vi "Test.vi"() -> ()   [LabVIEW 2019]
uses:
  VoiceCommandState.ctl
  <vilib>/myRIO/Instrument Drivers/Onboard IO/DIO/typedefs/DIO Reference.ctl
  <vilib>/myRIO/Common/Instrument Driver Framework/Utilities/typedefs/myRIO Generic Hardware Reference.ctl
  <vilib>/myRIO/Common/Instrument Driver Framework/Utilities/typedefs/Hardware Version Enum.ctl
  <vilib>/myRIO/Common/Instrument Driver Framework/Utilities/typedefs/myRIO v1.0 Reference.ctl
  <vilib>/myRIO/Common/Instrument Driver Framework/Utilities/typedefs/Generic FPGA Reference.ctl
  <vilib>/myRIO/Common/Instrument Driver Framework/myRIO v1.0/DIO/typedefs/DIO Channels List.ctl
  <vilib>/myRIO/Common/Instrument Driver Framework/myRIO v1.0/DIO/typedefs/DIO Channels Enum.ctl
  <vilib>/userDefined/High Color/nirio_resource_hc.ctl
  <vilib>/myRIO/Common/Instrument Driver Framework/Utilities/vis/Is FPGA Ref Available.vi
  <vilib>/myRIO/Common/Instrument Driver Framework/myRIO v1.0/DIO/vis/myRIO v1.1 Open DIO.vi
  <vilib>/myRIO/Common/Instrument Driver Framework/Utilities/vis/Validate Channels.vi
  <vilib>/myRIO/Common/Instrument Driver Framework/myRIO v1.0/DIO/vis/myRIO v1.0 Reserve DIO.vi
  <vilib>/myRIO/Common/Instrument Driver Framework/myRIO v1.0/UART/vis/myRIO v1.0 Close UART.vi
  <vilib>/myRIO/Common/Instrument Driver Framework/myRIO v1.0/Resource Manager/vis/myRIO v1.0 Reserve Channel List.vi
  <vilib>/myRIO/Common/Instrument Driver Framework/myRIO v1.0/DIO/vis/myRIO v1.0 Build MUX Configuration DIO.vi
  <vilib>/myRIO/Common/Instrument Driver Framework/myRIO v1.0/Resource Manager/vis/myRIO v1.0 Reserve Channel.vi
  <vilib>/myRIO/Common/Instrument Driver Framework/myRIO v1.0/Resource Manager/vis/myRIO v1.0 Unreserve Channel.vi
  <vilib>/myRIO/Common/Instrument Driver Framework/myRIO v1.0/Resource Manager/vis/myRIO v1.0 Create Configuration List.vi
  <vilib>/myRIO/Common/Instrument Driver Framework/myRIO v1.0/Resource Manager/vis/myRIO v1.0 Build Mutex Name.vi
  <vilib>/Utility/VariantDataType/GetNumericInfo.vi
  <vilib>/Utility/error.llb/Error Cluster From Error Code.vi
  <vilib>/myRIO/Common/Instrument Driver Framework/myRIO v1.0/myRIO v1.1 Open.vi
  <vilib>/myRIO/Common/Instrument Driver Framework/Utilities/vis/IO Manager.vi
  <vilib>/myRIO/Common/Instrument Driver Framework/Utilities/vis/Configuration Manager.vi
  <vilib>/myRIO/Common/Instrument Driver Framework/myRIO v1.0/Resource Manager/vis/myRIO v1.0 Configure IO.vi
  <vilib>/myRIO/Common/Instrument Driver Framework/myRIO v1.0/myRIO v1.0 Close.vi
  <vilib>/myRIO/Common/Instrument Driver Framework/myRIO v1.0/DIO/vis/myRIO v1.0 Write DIO.vi
  <vilib>/myRIO/Common/Instrument Driver Framework/Utilities/vis/FPGA Ref Manager.vi
  <vilib>/myRIO/Common/Instrument Driver Framework/myRIO v1.0/myRIO v1.0 Reset FPGA.vi
  <vilib>/myRIO/Common/Instrument Driver Framework/myRIO v1.0/IRQ/vis/myRIO v1.0 IRQ Info FGV.vi
  <vilib>/myRIO/Common/Instrument Driver Framework/myRIO v1.0/IRQ/vis/myRIO v1.0 Timer IRQ Info FGV.vi
  <vilib>/myRIO/Common/Instrument Driver Framework/myRIO v1.0/IRQ/vis/myRIO v1.0 ISR Agent.vi
  <vilib>/myRIO/Instrument Drivers/Utilities/vis/Reset Index.vi
  <vilib>/myRIO/Common/Instrument Driver Framework/myRIO v1.0/Resource Manager/vis/myRIO v1.0 Block Write Resource Manager.vi
  <vilib>/myRIO/Express VI/Onboard IO/DO/DO Express VI.xnode
  <vilib>/myRIO/Instrument Drivers/Onboard IO/DIO/vis/myRIO DIO Open.xnode
  Downloads/builds/DFRobot_ASR_myRIO_Lib/myRIO-1900/DFR_ISRM_myRIO/home/lvuser/natinst/bin/DFR_ISRM_myRIO.lvlibp
  Simple Queue Message/Simple Queue Message.lvlib
  <vilib>/myRIO/Instrument Drivers/Onboard IO/DIO/DIO.lvlib
  <vilib>/myRIO/Instrument Drivers/Utilities/Utilities.lvlib
panel:
  out "appended array 2":T1[](array[typedef])
  out "concatenated string":string
  out "String":string
  out "State":T1
  out "appended array":i32[](array[numeric])
  out "Result History":i32[](array[numeric])
  in  "Stop Button":bool
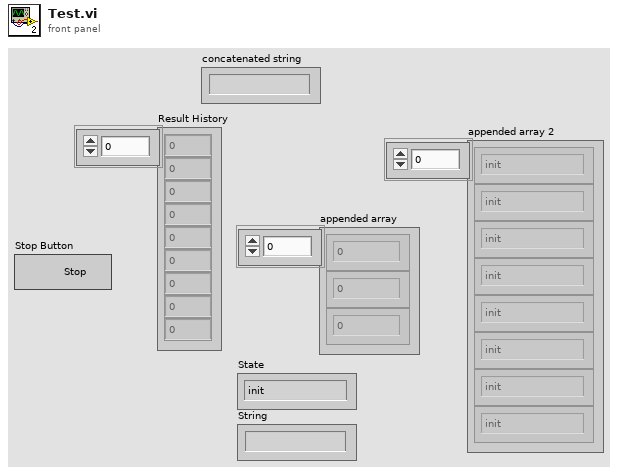
[diagram p1: front panel]
types:
  T1 = typedef "VoiceCommandState.ctl" = enum16{"init", "command", "quantity", "finish", "err"}
  T2 = typedef "DIO.lvlib/DIO Reference.ctl" = cluster{"myRIO Reference":T3, "DIO Channels List":T7}
  T3 = typedef "myRIO Generic Hardware Reference.ctl" = cluster{"myRIO Model":T4, "myRIO Hardware Reference":T5}
  T4 = typedef "Hardware Version Enum.ctl" = enum16{"Unknown", "myRIO-1900", "myRIO-1950", "roboRIO", "NI ELVIS RIO CM", "ELVIS III"}
  T5 = typedef "myRIO v1.0 Reference.ctl" = cluster{"Generic FPGA Reference":T6, "Allow multiple opens":bool}
  T6 = typedef "Generic FPGA Reference.ctl" = refnum<k20>
  T7 = typedef "DIO Channels List.ctl" = T8[]
  T8 = typedef "DIO Channels Enum.ctl" = enum16{"Not Connected", "C/DIO0", "C/DIO1", "C/DIO2", "C/DIO3", "C/DIO4", "C/DIO5", "C/DIO6", "C/DIO7", "A/DIO0", "A/DIO1", "A/DIO2", "A/DIO3", "A/DIO4", "A/DIO5", "A/DIO6", "A/DIO7", "A/DIO8", "A/DIO9", "A/DIO10", "A/DIO11", "A/DIO12", "A/DIO13", "A/DIO14", "A/DIO15", "A/DIO16", "A/DIO17", "A/DIO18", "A/DIO19", "B/DIO0", "B/DIO1", "B/DIO2", "B/DIO3", "B/DIO4", "B/DIO5", "B/DIO6", "B/DIO7", "B/DIO8", "B/DIO9", "B/DIO10", "B/DIO11", "B/DIO12", "B/DIO13", "B/DIO14", "B/DIO15", "B/DIO16", "B/DIO17", "B/DIO18", "B/DIO19", "LED0", "LED1", "LED2", "LED3", "Button0", "DIO/DIO0", "DIO/DIO1", "DIO/DIO2", "DIO/DIO3", "DIO/DIO4", "DIO/DIO5", "DIO/DIO6", "DIO/DIO7", "DIO/DIO8", "DIO/DIO9", "SPI/CS0", "SPI/CS1", "SPI/CS2", "SPI/CS3", "LED RADIO (Green)", "LED RADIO (Red)", "LED COMM (Green)", "LED COMM (Red)", "LED MODE (Green)", "LED MODE (Red)"}
  T9 = typedef "nirio_resource_hc.ctl" = tag
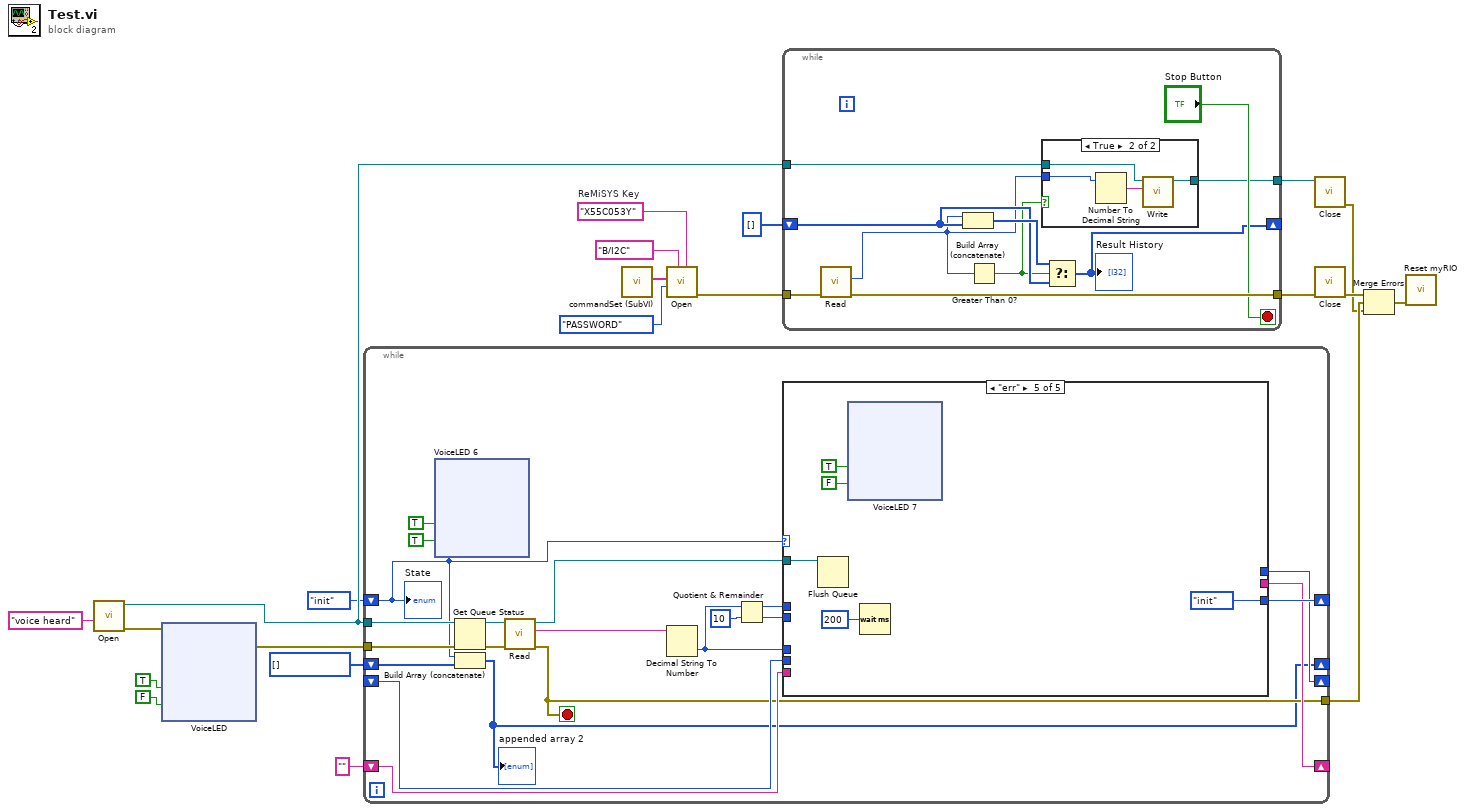
[diagram p0: block diagram]
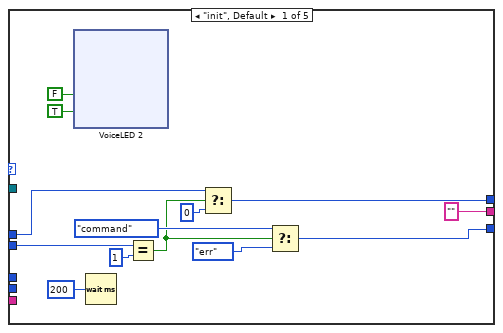
[diagram p2: hidden frame]
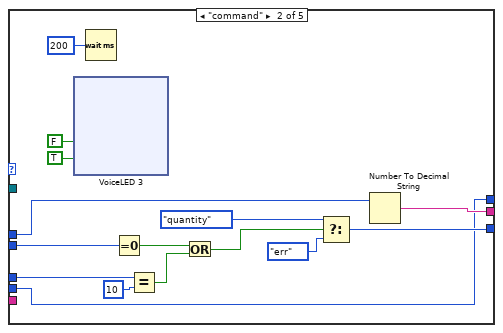
[diagram p3: hidden frame]
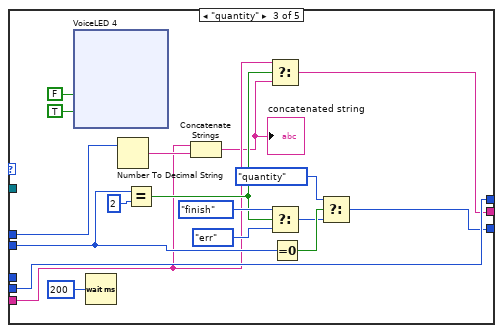
[diagram p4: hidden frame]
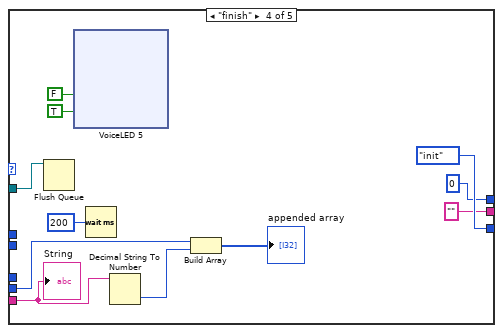
[diagram p5: hidden frame]
diagram:
  w2 = T1[] [] items=["init", "command", "quantity", "finish", "err"]
  w21 = "X55C053Y"  # ReMiSYS Key
  n1 = call "Open.vi"("name (unnamed)"="voice heard") -> ("error out"=w8:errorcluster, "queue out"=w13:refnum<queue>)  [unwired: 9 in]
  n2 = xnode "VoiceLED"("Green (C/DIO6 (DIO6))"=TRUE, "Red (C/DIO7 (DIO7))"=FALSE, "error in (no error)"=w8) -> ("error out"=w11:errorcluster)
  n3 = while {
    tunnel: w13 -> [w32]
    shift-right: [w41] -> _
    shift-left: VoiceCommandState."init" -> [w27]
    shift-right: [w38] -> _
    shift-left: "" -> [w37]
    tunnel: w11 -> [w30]
    shift-right: [w35] -> _
    shift-left: _ -> [w34]
    tunnel: [w28] -> w4
    shift-right: [w26] -> _
    shift-left: w2 -> [w25]
    stop <- w28 stop-if-true
    n4 = xnode "VoiceLED 6"("Green (C/DIO6 (DIO6))"=TRUE, "Red (C/DIO7 (DIO7))"=TRUE) -> ()  [unwired: 1 in, 1 out]
    n5 = Get Queue Status(queue=w32, error in (no error)=w30) -> (queue out=w31:refnum<queue>, error out=w29:errorcluster)  [unwired: 1 in, 6 out]
    n6 = Build Array (concatenate)(w27, w25) -> (w26:T1[])
    "appended array 2" <- w26
    n7 = call "Read.vi"("error in (no error)"=w29, "queue"=w31) -> ("error out"=w28:errorcluster, "state"=w42:string, "queue out"=w33:refnum<queue>)  [unwired: 6 in, 1 out]
    n8 = Decimal String To Number(string=w42) -> (number=w24:i32)  [unwired: 2 in, 1 out]
    n9 = Quotient & Remainder(x=w24, y=10) -> (x-y*floor(x/y)=w36:i32, floor(x/y)=w39:i32)
    n10 = case shown="\"err\"" w27 {
      tunnel: [w88 w142 w185 VoiceCommandState."init" VoiceCommandState."init"] -> w41
      tunnel: w39 -> [w87 w135 w193 _ _]
      tunnel: ["" w139 w181 "" _] -> w38
      tunnel: w37 -> [_ _ w183 w242 _]
      tunnel: [w82 w136 w186 0 ("f") _] -> w35
      tunnel: w36 -> [w83 w134 w180 _ _]
      tunnel: w34 -> [_ w136 w186 w243 _]
      tunnel: w33 -> [_ _ _ w234 w284]
      tunnel: w24 -> [_ w132 _ _ _]
      frame "init", Default {
        n11 = xnode "VoiceLED 2"("Green (C/DIO6 (DIO6))"=FALSE, "Red (C/DIO7 (DIO7))"=TRUE) -> ()  [unwired: 1 in, 1 out]
        n12 = Wait (ms)(milliseconds to wait=u32 200) -> ()  [unwired: 1 out]
        n13 = Equal?(x=w87, y=1) -> (x = y?=w84:bool)
        n14 = Select(t=w83, s=w84, f=0) -> (s? t:f=w82:i32)
        n15 = Select(t=VoiceCommandState."command", s=w84, f=VoiceCommandState."err") -> (s? t:f=w88:T1)
      }
      frame "command" {
        n16 = xnode "VoiceLED 3"("Green (C/DIO6 (DIO6))"=FALSE, "Red (C/DIO7 (DIO7))"=TRUE) -> ()  [unwired: 1 in, 1 out]
        n17 = Wait (ms)(milliseconds to wait=u32 200) -> ()  [unwired: 1 out]
        n18 = Equal To 0?(x=w135) -> (x = 0?=w133:bool)
        n19 = Equal?(x=w132, y=10) -> (x = y?=w130:bool)
        n20 = Or(x=w133, y=w130) -> (x .or. y?=w129:bool)
        n21 = Select(t=VoiceCommandState."quantity", s=w129, f=VoiceCommandState."err") -> (s? t:f=w142:T1)
        n22 = Number To Decimal String(number=w134) -> (decimal integer string=w139:string)  [unwired: 1 in]
      }
      frame "quantity" {
        n23 = xnode "VoiceLED 4"("Green (C/DIO6 (DIO6))"=FALSE, "Red (C/DIO7 (DIO7))"=TRUE) -> ()  [unwired: 1 in, 1 out]
        n24 = Wait (ms)(milliseconds to wait=u32 200) -> ()  [unwired: 1 out]
        n25 = Number To Decimal String(number=w180) -> (decimal integer string=w196:string)  [unwired: 1 in]
        n26 = Equal?(x=w193, y=2) -> (x = y?=w184:bool)
        n27 = Concatenate Strings(w183, w196) -> (w182:string)
        "concatenated string" <- w182
        n28 = Select(t=w183, s=w184, f=w182) -> (s? t:f=w181:string)
        n29 = Select(t=VoiceCommandState."finish", s=w184, f=VoiceCommandState."err") -> (s? t:f=w188:T1)
        n30 = Equal To 0?(x=w193) -> (x = 0?=w195:bool)
        n31 = Select(t=VoiceCommandState."quantity", s=w195, f=w188) -> (s? t:f=w185:T1)
      }
      frame "finish" {
        n32 = Flush Queue(queue=w234) -> ()  [unwired: 1 in, 3 out]
        n33 = xnode "VoiceLED 5"("Green (C/DIO6 (DIO6))"=FALSE, "Red (C/DIO7 (DIO7))"=TRUE) -> ()  [unwired: 1 in, 1 out]
        n34 = Wait (ms)(milliseconds to wait=u32 200) -> ()  [unwired: 1 out]
        n35 = Decimal String To Number(string=w242) -> (number=w241:i32)  [unwired: 2 in, 1 out]
        n36 = Build Array(w243, w241) -> (→"appended array":i32[])
        "String" <- w242
      }
      frame "err" {
        n37 = Flush Queue(queue=w284) -> ()  [unwired: 1 in, 3 out]
        n38 = xnode "VoiceLED 7"("Green (C/DIO6 (DIO6))"=TRUE, "Red (C/DIO7 (DIO7))"=FALSE) -> ()  [unwired: 1 in, 1 out]
        n39 = Wait (ms)(milliseconds to wait=u32 200) -> ()  [unwired: 1 out]
      }
    }
    "State" <- w27
  }
  n40 = call "commandSet (SubVI).vi"() -> ("CommandSet"=w1:string[])  [unwired: 11 in]
  n41 = call "Open.vi"("ReMiSYS Key"=w21, "Channel Name"=tag "B/I2C", "eMode"=enum16{"LOOP", "PASSWORD", "BUTTON"}."PASSWORD", "Command"=w1) -> ("error out"=w20:errorcluster)  [unwired: 7 in]
  n42 = while {
    tunnel: w20 -> [w330]
    tunnel: [w329] -> w17
    shift-right: [w326] -> _
    shift-left: i32[] [] -> [w325]
    tunnel: w13 -> [w324]
    tunnel: [w323] -> w14
    stop <- "Stop Button" stop-if-true
    n43 = call "Read.vi"("error in (no error)"=w330) -> ("error out"=w329:errorcluster, "Result out"=w321:i32)  [unwired: 9 in]
    n44 = Build Array (concatenate)(w321, w325) -> (w327:i32[])
    n45 = Greater Than 0?(x=w321) -> (x > 0?=w322:bool)
    n46 = case shown="True" w322 {
      tunnel: w324 -> [w331 w335]
      tunnel: [w331 w334] -> w323
      tunnel: w321 -> [_ w333]
      frame False {
      }
      frame True {
        n47 = Number To Decimal String(number=w333) -> (decimal integer string=w332:string)  [unwired: 1 in]
        n48 = call <vilib>:"Write.vi"("state"=w332, "queue"=w335) -> ("queue out"=w334:refnum<queue>)  [unwired: 8 in, 1 out]
      }
    }
    n49 = Select(t=w327, s=w322, f=w325) -> (s? t:f=w326:i32[])
    "Result History" <- w326
  }
  n50 = call "Close.vi"("queue out"=w14) -> ("error out"=w3:errorcluster)  [unwired: 10 in]
  n51 = call "Close.vi"("error in (no error)"=w17) -> ("error out"=w7:errorcluster)  [unwired: 10 in]
  n52 = Merge Errors(w7, w4, w3) -> (w6:errorcluster)
  n53 = call <vilib>:"Reset myRIO.vi"("error in (no error)"=w6) -> ()  [unwired: 10 in, 1 out]
